vi "Add CIPC Error Core.vi"(8 "error in (no error)":errorcluster, 10 "String to Append":string, 11 "Error":T1) -> (0 "error out":errorcluster)   [LabVIEW 2021, in "CIF_NI_CIPC.lvlib"]
doc: "This VI is set for non-reentrant execution to optimize memory. This core will only be called in an error case when jitter does not matter."
uses:
  CIF_NI_CIPC.lvlib
  TypeDefs/Errors.ctl
  <vilib>/CIF Foundation/CIF Utilities/Errors/Errors_CIF_U.lvlib
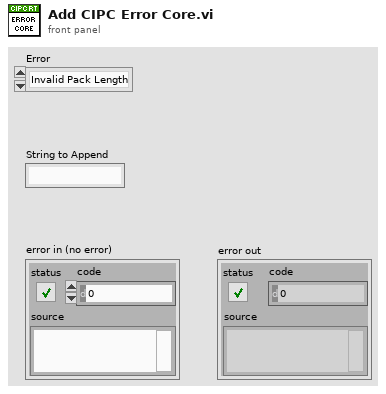
[diagram p1: front panel]
types:
  T1 = typedef "CIF_NI_CIPC.lvlib/Errors.ctl" = enum16{"Invalid Pack Length", "Invalid Pack Destination", "Unsupported Type", "Missing Library"}
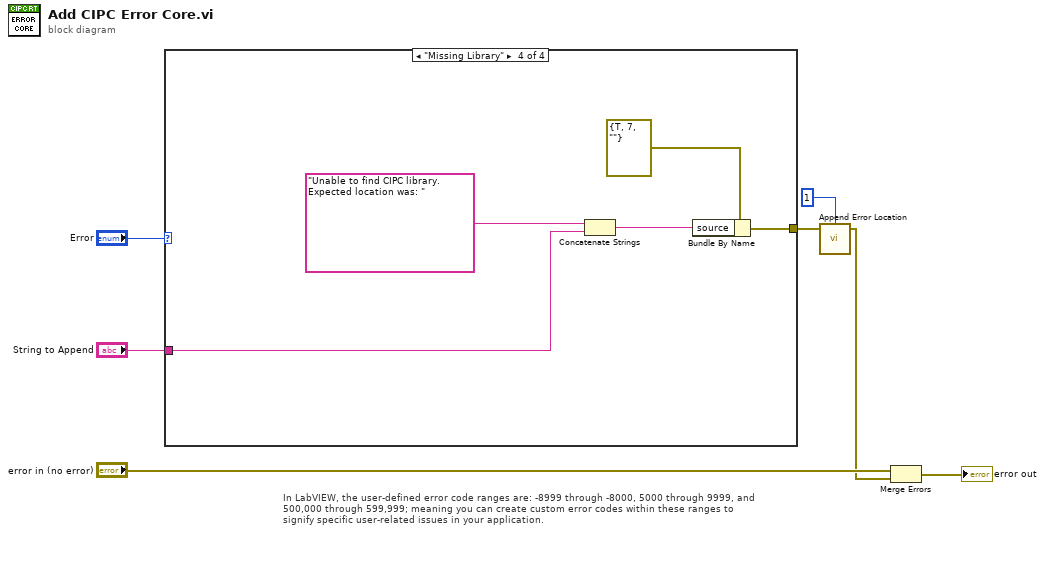
[diagram p0: block diagram]
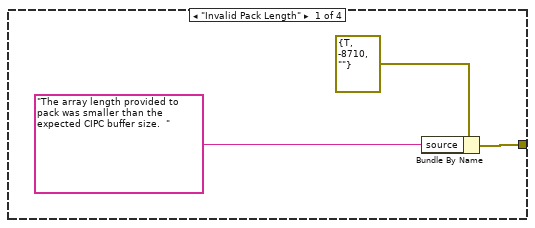
[diagram p2: hidden frame]
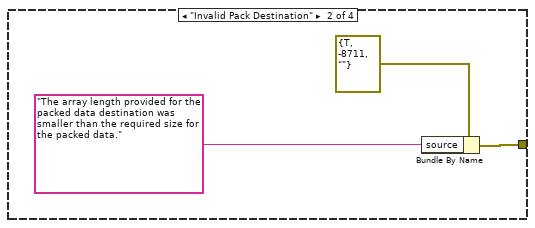
[diagram p3: hidden frame]
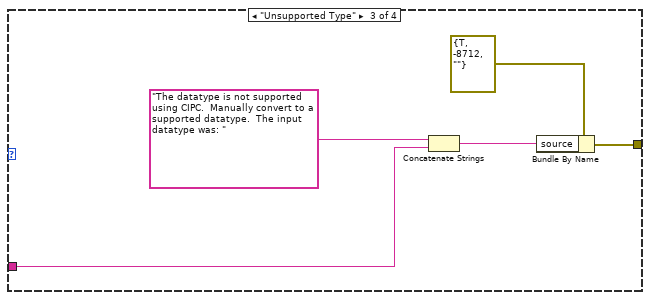
[diagram p4: hidden frame]
diagram:
  # "In LabVIEW, the user-defined error code ranges are: -8999 through -8000, 5000 through 9999, and 500,000 through 599,999; meaning you can create custom error codes within these ranges to signify specific user-related issues in your application."
  n1 = case shown="\"Missing Library\"" "Error" {
    tunnel: "String to Append" -> [_ _ w14 w19]
    tunnel: [w9 w12 w17 w22] -> w7
    frame "Invalid Pack Length" {
      n2 = Bundle By Name(cluster=errorcluster {"status"=TRUE, "code"=-8710, "source"=""} ("Invalid ID"), "source"="The array length provided to pack was smaller than the expected CIPC buffer size.  ") -> (w9:errorcluster)
    }
    frame "Invalid Pack Destination" {
      n3 = Bundle By Name(cluster=errorcluster {"status"=TRUE, "code"=-8711, "source"=""} ("Invalid ID"), "source"="The array length provided for the packed data destination was smaller than the required size for the packed data.") -> (w12:errorcluster)
    }
    frame "Unsupported Type" {
      n4 = Concatenate Strings("The datatype is not supported using CIPC.  Manually convert to a supported datatype.  The input datatype was: " ("source"), w14) -> (w15:string)
      n5 = Bundle By Name(cluster=errorcluster {"status"=TRUE, "code"=-8712, "source"=""} ("Invalid ID"), "source"=w15) -> (w17:errorcluster)
    }
    frame "Missing Library" {
      n6 = Concatenate Strings("Unable to find CIPC library.  Expected location was: " ("source"), w19) -> (w20:string)
      n7 = Bundle By Name(cluster=errorcluster {"status"=TRUE, "code"=7, "source"=""} ("Invalid ID"), "source"=w20) -> (w22:errorcluster)
    }
  }
  n8 = call <vilib>:"Append Error Location.vi"("error in (no error)"=w7, "Chain Depth"=1) -> ("error out"=w3:errorcluster)  [unwired: 3 in]
  n9 = Merge Errors("error in (no error)", w3) -> (→"error out":errorcluster)
